vi "FileIO-Validate Filepath.vi"(5 "Path In":path) -> (2 "Path Out":path)   [LabVIEW 2015]
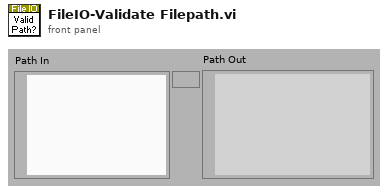
[diagram p1: front panel]
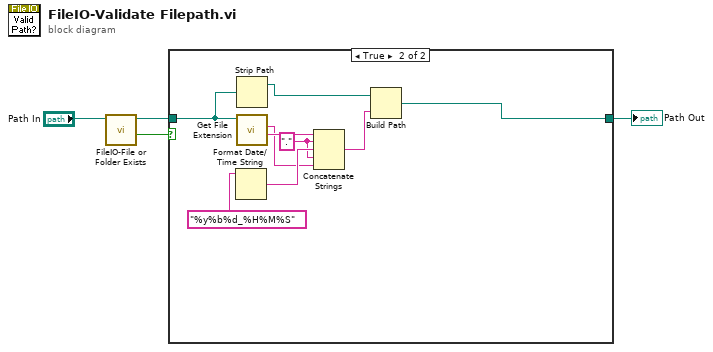
[diagram p0: block diagram]
diagram:
  n1 = call "FileIO-File or Folder Exists.vi"("path"="Path In") -> ("Exists?"=w2:bool, "dup path"=w3:path)  [unwired: 7 in, 2 out]
  n2 = case shown="True" w2 {
    tunnel: w3 -> [w5 w14]
    tunnel: [w5 w8] -> w1
    frame False {
    }
    frame True {
      w6 = "." ("string")
      n3 = Format Date/Time String(time format string (%c)="%y%b%d_%H%M%S") -> (date/time string=w11:string)  [unwired: 2 in]
      n4 = Strip Path(path=w14) -> (stripped path=w13:path)  [unwired: 1 out]
      n5 = call <vilib>:"Get File Extension.vi"("file"=w14) -> ("filename without extension"=w12:string, "lowercase file extension"=w10:string)  [unwired: 6 in, 3 out]
      n6 = Concatenate Strings(w12, w6, w11, w6, w10) -> (w9:string)
      n7 = Build Path(base path=w13, name or relative path=w9) -> (appended path=w8:path)
    }
  }
  "Path Out" <- w1
